vi "int random.vi"() -> ()   [LabVIEW 2018, in "LV2Julia_core.lvlib"]
uses:
  LV2Julia_core.lvlib
panel:
  out "rnd":i16
  out "span":dbl
  out "min":dbl format="%.2f"
  out "max":dbl format="%.2f"
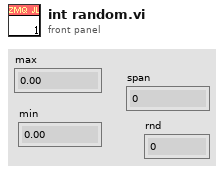
[diagram p1: front panel]
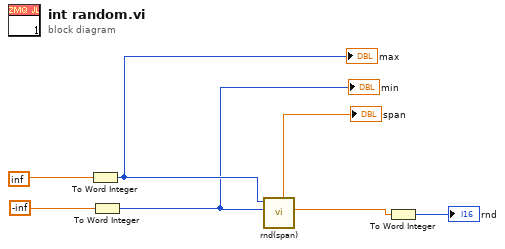
[diagram p0: block diagram]
diagram:
  n1 = To Word Integer(number=inf) -> (16bit integer=w5:i16)
  "max" <- w5
  n2 = To Word Integer(number=-inf) -> (16bit integer=w2:i16)
  "min" <- w2
  n3 = call "rnd(span).vi"("min"=w2, "max"=w5) -> ("mapped"=w3:dbl, "span"=→"span":dbl)  [unwired: 8 in]
  n4 = To Word Integer(number=w3) -> (16bit integer=→"rnd":i16)
